vi "Validate.vi"(8 "error in (no error)":errorcluster, 11 "Project Action Interface in":refnum<class>) -> (0 "error out":errorcluster, 1 "Valid?":bool, 3 "Project Action Interface out":refnum<class>)   [LabVIEW 2020, in "ProjectBuilder.lvlib" / "Project Action Interface.lvclass"]
uses:
  Project Action Interface.lvclass
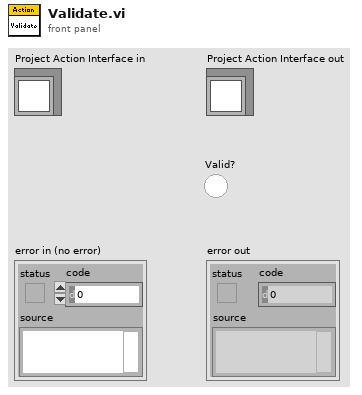
[diagram p1: front panel]
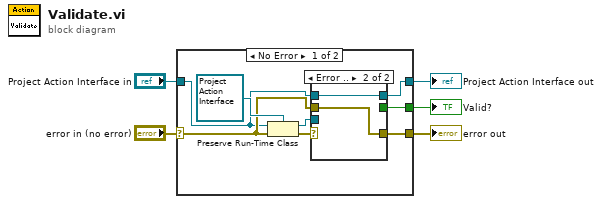
[diagram p0: block diagram]
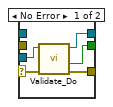
[diagram p2: hidden frame]
diagram:
  n1 = case shown="No Error" "error in (no error)" {
    selector: "error in (no error)" -> [w7 w22]
    tunnel: [w13 w22] -> w4
    tunnel: [w12 w21] -> w2
    tunnel: "Project Action Interface in" -> [w6 w21]
    tunnel: [w11 _] -> w1
    frame No Error {
      n2 = Preserve Run-Time Class(object in=w6, error in=w7, 2:refnum<class "Project Action Interface.lvclass"> refnum ("ProjectBuilder.lvlib:Project Action Interface.lvclass")) -> (object out=w9:refnum<class "Project Action Interface.lvclass">, error out=w10:errorcluster)
      n3 = case shown="Error .." w10 {
        selector: w10 -> [w15 _]
        tunnel: [w18 w20] -> w13
        tunnel: [w17 w19] -> w12
        tunnel: [w16 _] -> w11
        tunnel: w9 -> [w14 _]
        tunnel: w7 -> [_ w20]
        tunnel: w6 -> [_ w19]
        frame No Error {
          n4 = call-dynamic "Validate_Do.vi"("error in (no error)"=w15, "Project Action Interface in"=w14) -> ("error out"=w18:errorcluster, "Valid?"=w16:bool, "Project Action Interface out"=w17:refnum<class "Project Action Interface.lvclass">)  [unwired: 7 in]
        }
        frame Error {
        }
      }
    }
    frame Error {
    }
  }
  "error out" <- w4
  "Project Action Interface out" <- w2
  "Valid?" <- w1
